vi "Queue.vi"(0 "Cluster":T2, 1 "Override Build\nFile Write":bool, 2 "percentage of random uncertainty allowed":dbl=5.0 format="%#_13g", 3 "Uncertainty Contributions":dbl[](array[numeric]), 5 "Saving Cluster":T1, 7 "Collect Transient":bool, 9 "Save Data":bool, 11 "Data In":dbl[](array[numeric]), 12 "units":string(combo), 13 "file path (dialog if empty)":path=path "C:/Users/betsrgadmin/Desktop/80_Labview/80_Ton_Labview/test_matrix.csv", 14 "Tester":string, 15 "Loop Iter":i32) -> (4 "queue out":refnum<queue>, 6 "Number in Queue":i32, 10 "Numeric":i32)   [LabVIEW 2017]
doc: "This VI takes the data that is being collected in the host VI and does three things.\n1. Determines the steadiness of the data and automatically saves the data when steadiness has been achieved, if the user decides to use this function.\n2. Saves the data into a raw data file and a build file. The raw data file contains every point that is collected for the test. The build file contains the average values for each variable over the duration of the test.\n3. Loops through the test matrix if the user decides to use that function."
uses:
  <vilib>/Analysis/baseanly.llb/Mean (DBL).vi
  98cf6813-202c-4cae-8cd8-e25b1f3a8822.vi
  <vilib>/Analysis/NI_AALBase.lvlib
panel:
  in  "Steady Indicator":bool=TRUE
  out "Raw Data Array":dbl[][](array[numeric])
  out "pre-arranged":dbl[][](array[numeric])
  out "Array of Averages for Build Sheet":dbl[](array[numeric])
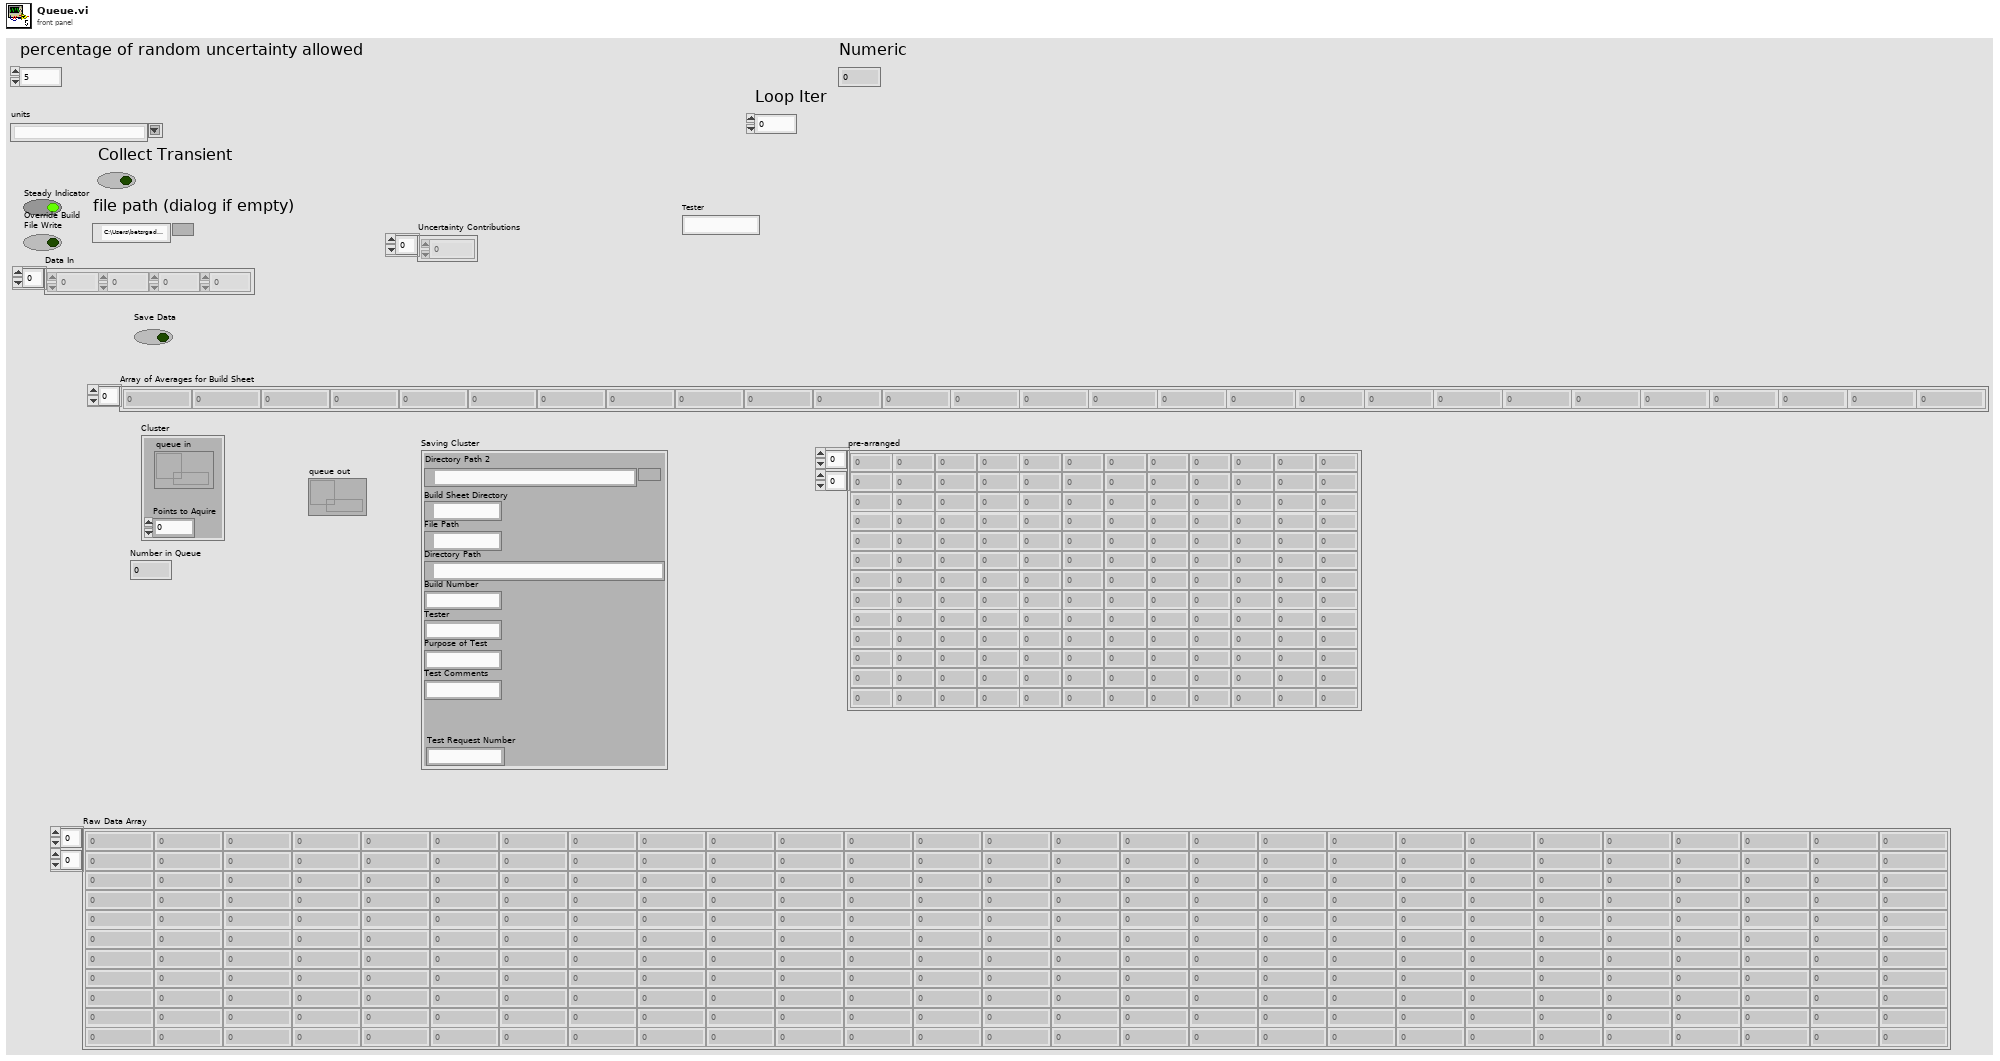
[diagram p1: front panel]
types:
  T1 = cluster{"Build Sheet Directory":path, "File Path":path, "Directory Path":path, "Build Number":string, "Tester":string, "Purpose of Test":string, "Test Comments ":string, "Test Request Number":string, "Directory Path 2":path}
  T2 = cluster{"queue in":refnum<queue>, "Points to Aquire":i32}
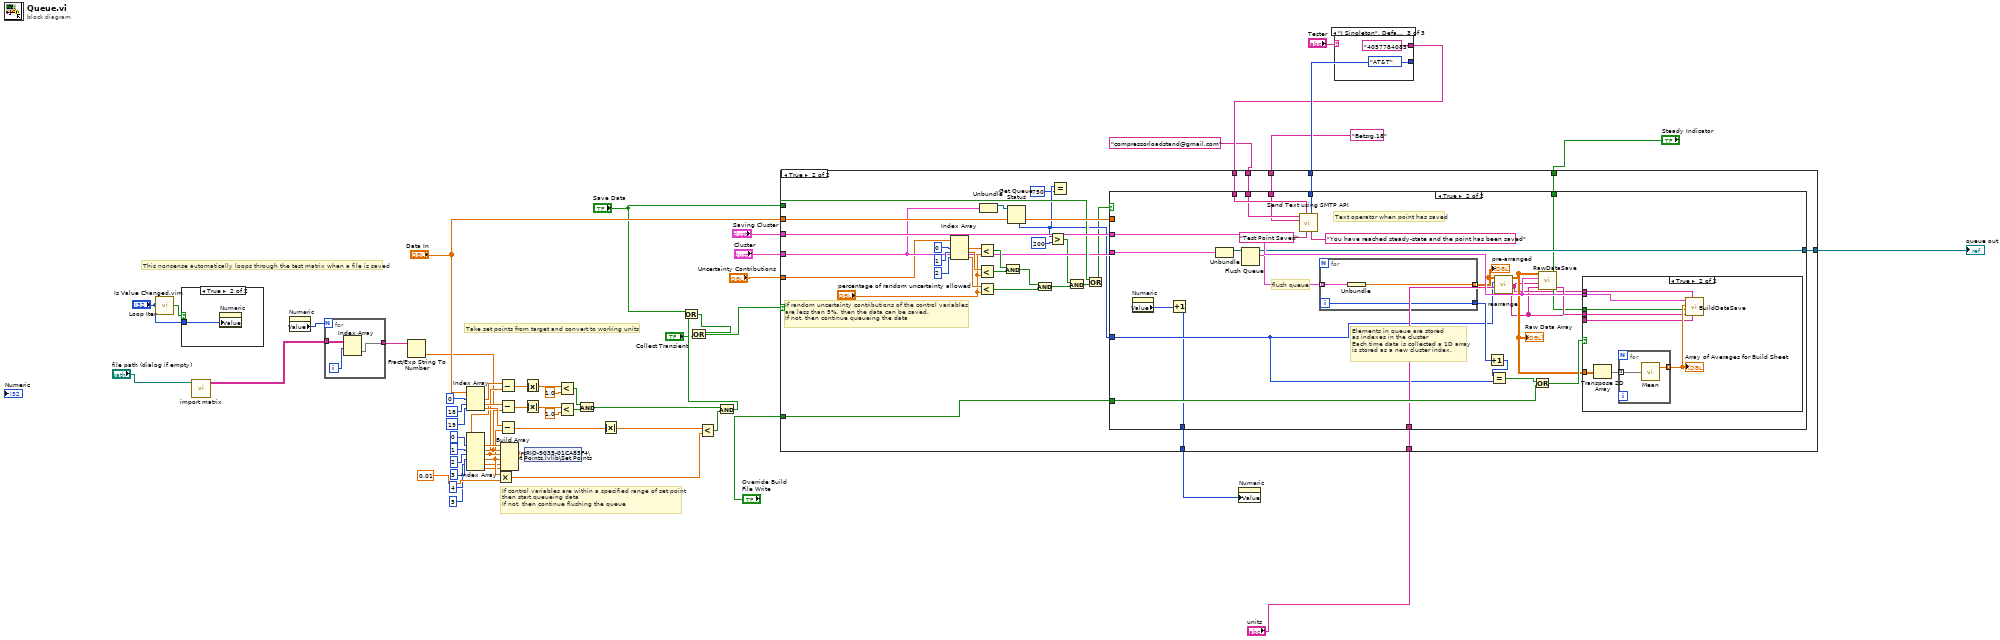
[diagram p0: block diagram]
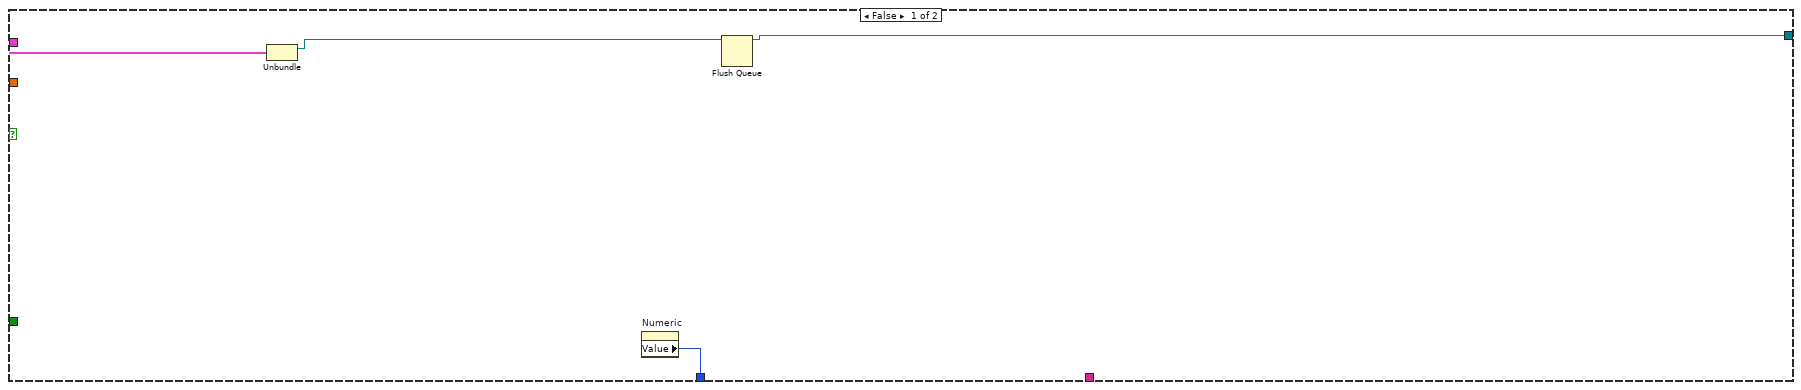
[diagram p3: hidden frame]
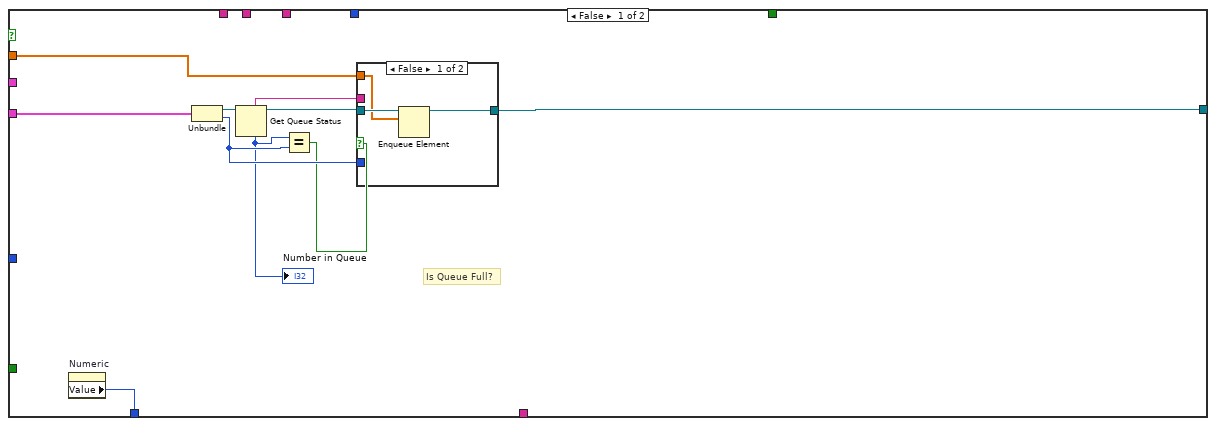
[diagram p4: hidden frame]
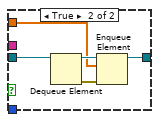
[diagram p5: hidden frame]
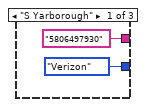
[diagram p7: hidden frame]
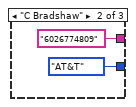
[diagram p8: hidden frame]
diagram:
  # "This nonsense automatically loops through the test matrix when a file is saved"
  # "If control variables are within a specified range of set point\nthen start queueing data\nIf not, then continue flushing the queue"
  # "Take set points from target and convert to working units"
  n1 = call "Is Value Changed.vim"("value"="Loop Iter") -> ("changed or first call?"=w15:bool)
  n2 = case shown="True" w15 {
    tunnel: "Loop Iter" -> [_ w60]
    frame False {
    }
    frame True {
      n3 = property on="Numeric" class="DigNum (strict)"("Value"=w60) -> ()  [unwired: 2 in, 2 out]
    }
  }
  n4 = call "import matrix.vi"("file path (dialog if empty)"="file path (dialog if empty)") -> ("String Array From File"=w59:string[][])  [unwired: 10 in]
  n5 = property on="Numeric" class="DigNum (strict)"() -> ("Value"=w13:i32)  [unwired: 2 in, 2 out]
  n6 = for {
    N: w13 -> [_]
    tunnel: w59 -> [w63]
    tunnel: [w62] -> w18
    i -> [w61]
    n7 = Index Array(array=w63, index (row)=w61) -> (element=w62:string[])  [unwired: 1 in]
  }
  n8 = Fract/Exp String To Number(string=w18) -> (number=w17:dbl[])  [unwired: 3 in, 1 out]
  n9 = Index Array(array="Data In", index #1=0 ("index"), index #2=18 ("index"), index #3=19 ("index")) -> (element #1=w42:dbl, element #2=w34:dbl, element #3=w29:dbl)
  n10 = Index Array(array=w17, index #1=0 ("index"), index #2=1 ("index"), index #3=2 ("index"), index #4=3 ("index"), index #5=4 ("index"), index #6=5 ("index")) -> (element #1=w22:dbl, element #2=w21:dbl, element #3=w20:dbl, element #4=w10:dbl, element #5=w2:dbl, element #6=w1:dbl)
  n11 = Multiply(x=w10, y=0.01) -> (x*y=w9:dbl)
  n12 = Subtract(x=w42, y=w20) -> (x-y=w41:dbl)
  n13 = Subtract(x=w34, y=w21) -> (x-y=w37:dbl)
  n14 = Subtract(x=w29, y=w10) -> (x-y=w31:dbl)
  n15 = Build Array(w22, w21, w20, w10, w2, w1) -> (w16:dbl[])
  n16 = Absolute Value(x=w41) -> (abs(x)=w40:dbl)
  n17 = Absolute Value(x=w37) -> (abs(x)=w36:dbl)
  n18 = shared-variable "NI-cRIO-9035-01CA85F4\\Set Points.lvlib\\Set Points"(w16) -> ()  [unwired: 1 in, 1 out]
  n19 = Less?(x=w40, y=1.0) -> (x < y?=w38:bool)
  n20 = Less?(x=w36, y=1.0) -> (x < y?=w33:bool)
  n21 = And(x=w38, y=w33) -> (x .and. y?=w32:bool)
  n22 = Absolute Value(x=w31) -> (abs(x)=w30:dbl)
  n23 = Less?(x=w30, y=w9) -> (x < y?=w28:bool)
  n24 = And(x=w32, y=w28) -> (x .and. y?=w19:bool)
  n25 = Or(x="Save Data", y=w19) -> (x .or. y?=w8:bool)
  n26 = Or(x=w8, y="Collect Transient") -> (x .or. y?=w7:bool)
  n27 = case shown="\"J Singleton\", Default" "Tester" {
    tunnel: [enum16{"T-Mobile", "AT&T", "Verizon", "Sprint"}."Verizon" ("Carrier") enum16{"T-Mobile", "AT&T", "Verizon", "Sprint"}."AT&T" ("Carrier") enum16{"T-Mobile", "AT&T", "Verizon", "Sprint"}."AT&T" ("Carrier")] -> w50
    tunnel: ["5806497930" ("phone number") "6026774809" ("phone number") "4057784085" ("phone number")] -> w49
    frame "S Yarborough" {
    }
    frame "C Bradshaw" {
    }
    frame "J Singleton", Default {
    }
  }
  n28 = case shown="True" w7 {
    tunnel: "Cluster" -> [w73 w88]
    tunnel: "Saving Cluster" -> [_ w106]
    tunnel: [w71 w105] -> w46
    tunnel: "Steady Indicator" -> [_ w104]
    tunnel: "Override Build\nFile Write" -> [_ w103]
    tunnel: "units" -> [_ w102]
    tunnel: "Data In" -> [_ w101]
    tunnel: "Save Data" -> [_ w100]
    tunnel: "Uncertainty Contributions" -> [_ w82]
    tunnel: w50 -> [_ w81]
    tunnel: w49 -> [_ w80]
    tunnel: "compressorloadstand@gmail.com" ("Email") -> [_ w79]
    tunnel: "Betsrg.18" ("Password") -> [_ w78]
    tunnel: [w70 w77] -> w12
    frame False {
      n29 = Unbundle(w73) -> ("queue in"=w72:refnum<queue>)  [unwired: 1 out]
      n30 = property on="Numeric" class="DigNum (strict)"() -> ("Value"=w70:i32)  [unwired: 2 in, 2 out]
      n31 = Flush Queue(queue=w72) -> (queue out=w71:refnum<queue>)  [unwired: 1 in, 2 out]
    }
    frame True {
      # "If random uncertainty contributions of the control variables\nare less than 5%, then the data can be saved.\nIf not, then continue queueing the data"
      n32 = Index Array(array=w82, index #1=0 ("index"), index #2=1 ("index"), index #3=2 ("index")) -> (element #1=w96:dbl, element #2=w95:dbl, element #3=w94:dbl)
      n33 = Less?(x=w96, y="percentage of random uncertainty allowed") -> (x < y?=w92:bool)
      n34 = Less?(x=w95, y="percentage of random uncertainty allowed") -> (x < y?=w91:bool)
      n35 = Less?(x=w94, y="percentage of random uncertainty allowed") -> (x < y?=w89:bool)
      n36 = Unbundle(w88) -> ("queue in"=w87:refnum<queue>)  [unwired: 1 out]
      n37 = And(x=w92, y=w91) -> (x .and. y?=w90:bool)
      n38 = Get Queue Status(queue=w87) -> (# elements in queue=w76:i32)  [unwired: 1 in, 8 out]
      n39 = And(x=w90, y=w89) -> (x .and. y?=w85:bool)
      n40 = Greater?(x=w76, y=200) -> (0:w84:bool)
      n41 = Equal?(x=w76, y=750) -> ()  [unwired: 1 out]
      n42 = And(x=w84, y=w85) -> (x .and. y?=w83:bool)
      n43 = Or(x=w100, y=w83) -> (x .or. y?=w74:bool)
      n44 = case shown="True" w74 {
        tunnel: w88 -> [w115 w150]
        tunnel: w106 -> [_ w149]
        tunnel: [w109 w148] -> w105
        tunnel: w104 -> [_ w145]
        tunnel: w103 -> [_ w142]
        tunnel: w101 -> [w110 _]
        tunnel: w102 -> [_ w135]
        tunnel: w76 -> [_ w127]
        tunnel: w81 -> [_ w133]
        tunnel: w80 -> [_ w132]
        tunnel: w79 -> [_ w131]
        tunnel: w78 -> [_ w128]
        tunnel: [w107 w125] -> w77
        frame False {
          # "Is Queue Full?"
          n45 = property on="Numeric" class="DigNum (strict)"() -> ("Value"=w107:i32)  [unwired: 2 in, 2 out]
          n46 = Unbundle(w115) -> ("queue in"=w116:refnum<queue>, "Points to Aquire"=w114:i32)
          n47 = Get Queue Status(queue=w116) -> (queue out=w108:refnum<queue>, queue name=w111:string, # elements in queue=w113:i32)  [unwired: 1 in, 6 out]
          "Number in Queue" <- w113
          n48 = Equal?(x=w113, y=w114) -> (x = y?=w112:bool)
          n49 = case shown="False" w112 {
            tunnel: w114 -> [_ _]
            tunnel: w111 -> [_ _]
            tunnel: [w119 w122] -> w109
            tunnel: w108 -> [w118 w121]
            tunnel: w110 -> [w117 w120]
            frame False {
              n50 = Enqueue Element(queue=w118, element=w117) -> (queue out=w119:refnum<queue>)  [unwired: 1 in, 3 out]
            }
            frame True {
              n51 = Dequeue Element(queue=w121) -> (queue out=w124:refnum<queue>, error out=w123:errorcluster)  [unwired: 1 in, 3 out]
              n52 = Enqueue Element(queue=w124, element=w120, error in (no error)=w123) -> (queue out=w122:refnum<queue>)  [unwired: 3 out]
            }
          }
        }
        frame True {
          # "Text operator when point has saved"
          # "Elements in queue are stored\nas indexes in the cluster\nEach time data is collected a 1D array\nis stored as a new cluster index."
          # "flush queue"
          n53 = property on="Numeric" class="DigNum (strict)"() -> ("Value"=w126:i32)  [unwired: 2 in, 2 out]
          n54 = Increment(x=w126) -> (x+1=w125:i32)
          n55 = Unbundle(w150) -> ("queue in"=w134:refnum<queue>)  [unwired: 1 out]
          n56 = Flush Queue(queue=w134) -> (queue out=w148:refnum<queue>, remaining elements=w147:cluster{dbl[]}[])  [unwired: 1 in, 1 out]
          n57 = call "Send Text using SMTP API.vi"("Body"="You have reached steady-state and the point has been saved", "Carrier"=w133, "Subject"="Test Point Saved", "phone number"=w132, "Password"=w128, "Email"=w131) -> ()  [unwired: 6 in]
          n58 = for {
            tunnel: [w163] -> w139 mode=indexing
            tunnel: w147 -> [w162] mode=indexing
            tunnel: [w161] -> w141
            i -> [w161]
            n59 = Unbundle(w162) -> (w163:dbl[])
          }
          "pre-arranged" <- w139
          n60 = Increment(x=w141) -> (x+1=w140:i32)
          n61 = Equal?(x=w140, y=w127) -> (x = y?=w143:bool)
          n62 = call "rearrange.vi"("units"=w135, "Points to Aquire"=w127, "Array in"=w139) -> ("units"=w136:string[], "varnames"=w137:string[], "Array out"=w138:dbl[][])  [unwired: 6 in]
          "Raw Data Array" <- w138
          n63 = Or(x=w143, y=w142) -> (x .or. y?=w144:bool)
          n64 = call "RawDataSave.vi"("units"=w136, "varnames"=w137, "Saving Cluster"=w149, "Array"=w138) -> ("raw data filename string"=w146:string)  [unwired: 7 in]
          n65 = case shown="True" w144 {
            tunnel: w149 -> [_ w158]
            tunnel: w138 -> [_ w155]
            tunnel: w146 -> [_ w154]
            tunnel: w137 -> [_ w153]
            tunnel: w136 -> [_ w152]
            tunnel: w145 -> [_ w151]
            frame False {
            }
            frame True {
              n66 = Transpose 2D Array(2D array=w155) -> (transposed array=w157:dbl[][])
              n67 = for {
                tunnel: w157 -> [w159] mode=indexing
                tunnel: [w160] -> w156 mode=indexing
                n68 = call-poly <vilib>:"Mean.vi"("X"=w159) -> ("mean"=w160:dbl)  [unwired: 1 out]
              }
              "Array of Averages for Build Sheet" <- w156
              n69 = call "BuildDataSave.vi"("units"=w152, "varnames"=w153, "raw data filename string"=w154, "Steady Indicator"=w151, "Array"=w156, "Saving Cluster"=w158) -> ()  [unwired: 6 in]
            }
          }
        }
      }
    }
  }
  "queue out" <- w46
  n70 = property on="Numeric" class="DigNum (strict)"("Value"=w12) -> ()  [unwired: 2 in, 2 out]
